vi "Main.vi"(8 "error in":errorcluster, 11 "System Monitor UI in":refnum<class "System Monitor UI.lvclass">) -> (0 "error out":errorcluster, 3 "System Monitor UI out":refnum<class "System Monitor UI.lvclass">)   [LabVIEW 2017, in "System Monitor UI.lvclass"]
doc: "The <b>Queued Message Handler</b> of the Worker that owns this VI."
uses:
  System Monitor UI.lvclass
  C:/Program Files (x86)/National Instruments/LabVIEW 2017/vi.lib/addons/_Workers/Library/Classes/Worker/Worker.lvclass
  Initialization Data.ctl
  Response Cases.ctl
  System Monitor UI.lvclass/System Monitor UI.ctl
  rwr_Get Main VI Ref.ctl
  rwr_Get Main VI Ref Reply.ctl
  rqp_Update cRIO System Data.ctl
  Shared/System Health Data.ctl
  <vilib>/addons/_Workers/Library/Classes/Message Queue/Message Queue.lvclass
panel:
  out "Total Virtual Memory (MB)":u32
  out "Total Physical Memory (MB)":u32
  out "Primary Hard Drive Capacity (MB)":u32
  out "Primary Hard Drive Available (MB)":dbl
  out "Hard Drive Space Used (%)":dbl(slide) scale=0.0..100.0
  out "Memory":dbl[][](graph)
  out "CPUs":u32[][](graph)
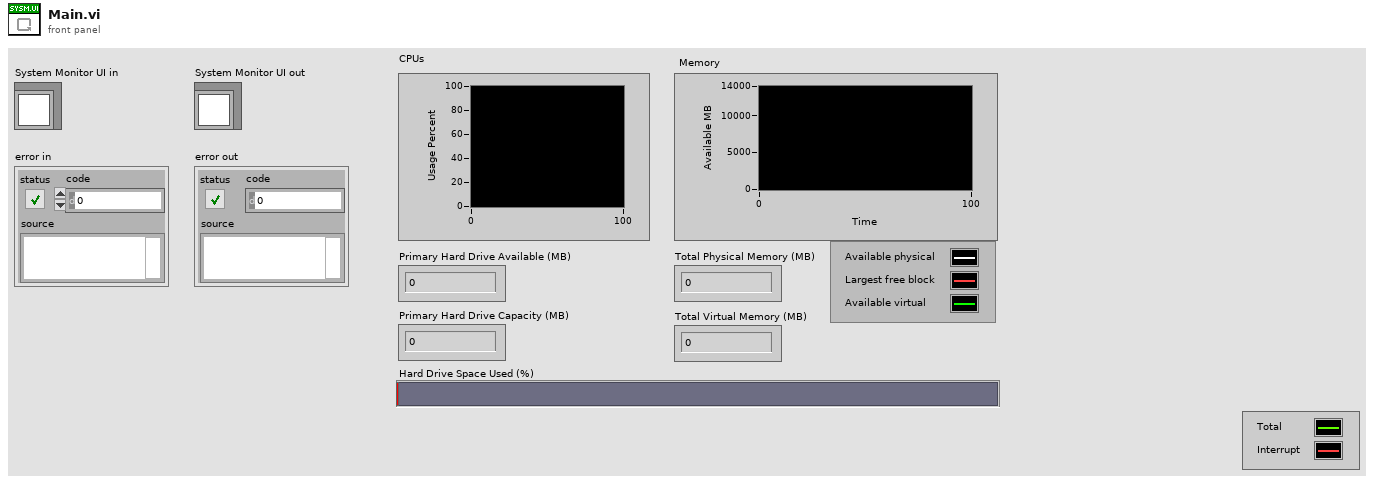
[diagram p1: front panel]
types:
  T1 = typedef "System Monitor UI.lvclass/Initialization Data.ctl" = cluster{"Response Cases":T2}
  T2 = typedef "System Monitor UI.lvclass/Response Cases.ctl" = cluster{"Placeholder - Can be deleted":string}
  T3 = typedef "System Monitor UI.lvclass/rwr_Get Main VI Ref Reply.ctl" = cluster{"Main VI Ref":refnum<vi>}
  T4 = typedef "System Monitor UI.lvclass/rwr_Get Main VI Ref.ctl" = cluster{"String":string}
  T5 = typedef "System Health Data.ctl" = cluster{"CPUs":u32[][], "Memory":dbl[][], "Hard Drive Space Used (%)":dbl, "Primary Hard Drive Available (MB)":dbl, "Primary Hard Drive Capacity (MB)":u32, "Total Physical Memory (MB)":u32, "Total Virtual Memory (MB)":u32}
  T6 = typedef "System Monitor UI.lvclass/rqp_Update cRIO System Data.ctl" = cluster{"Data as String":string}
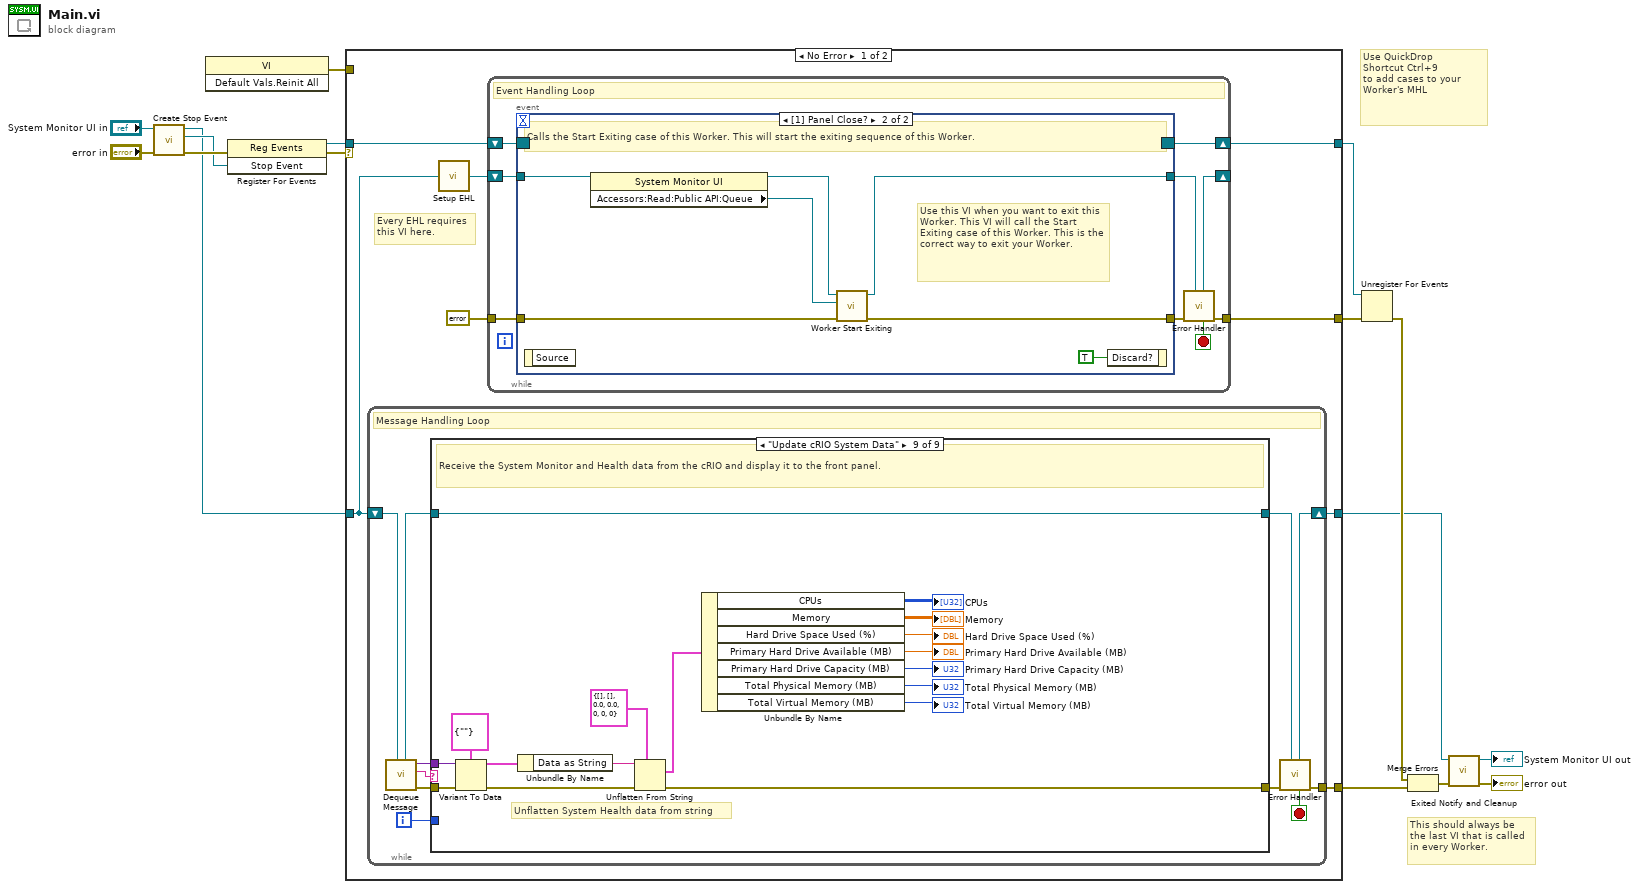
[diagram p0: block diagram]
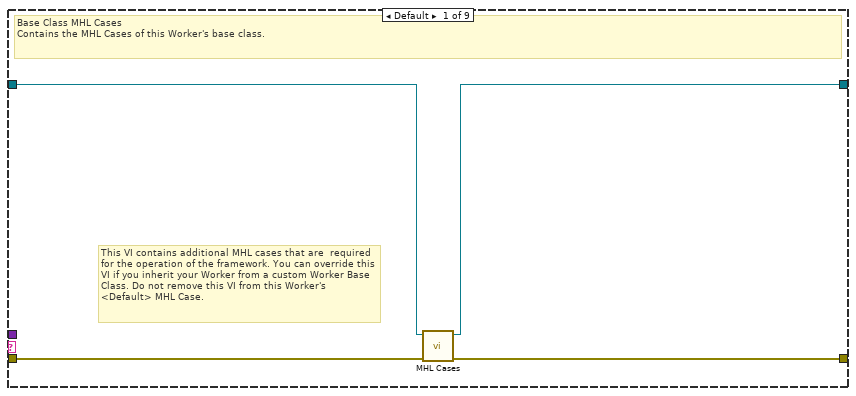
[diagram p2: hidden frame]
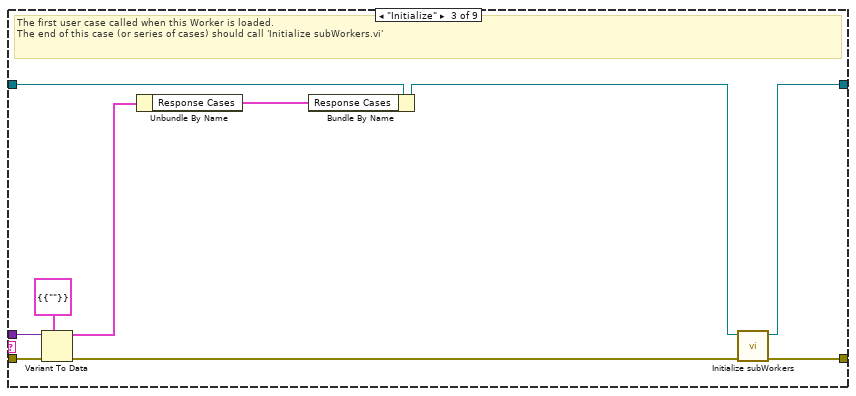
[diagram p4: hidden frame]
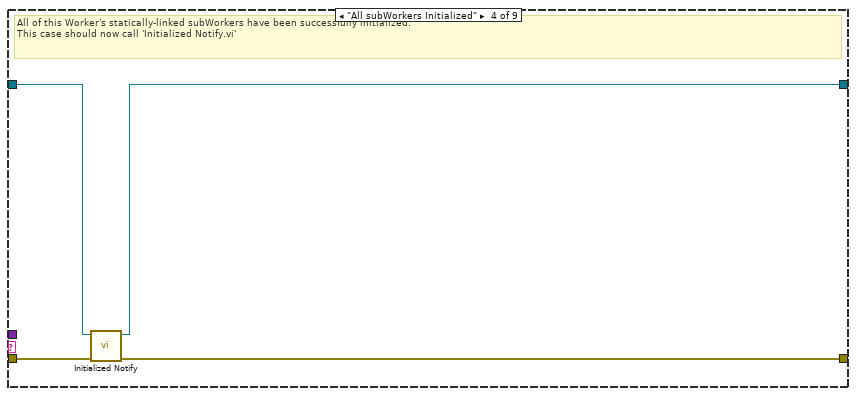
[diagram p5: hidden frame]
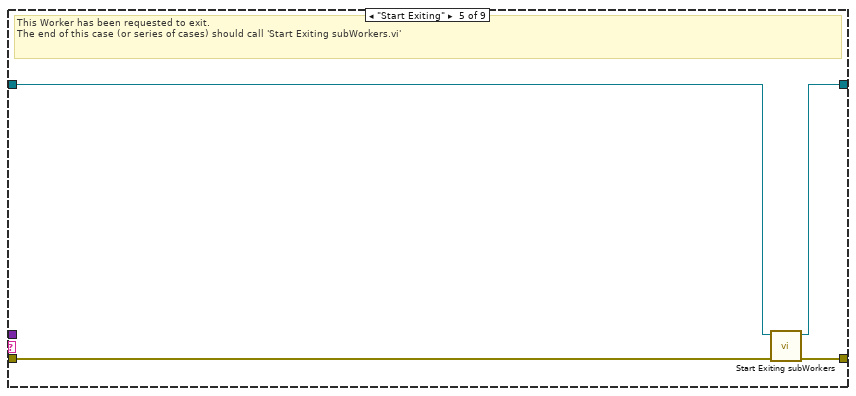
[diagram p6: hidden frame]
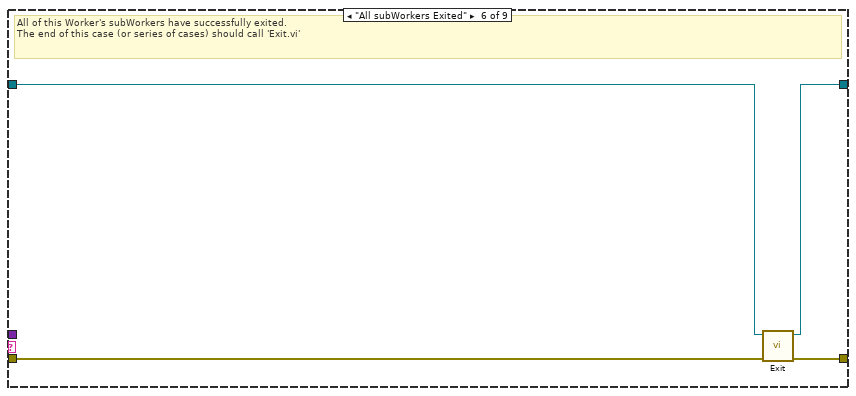
[diagram p7: hidden frame]
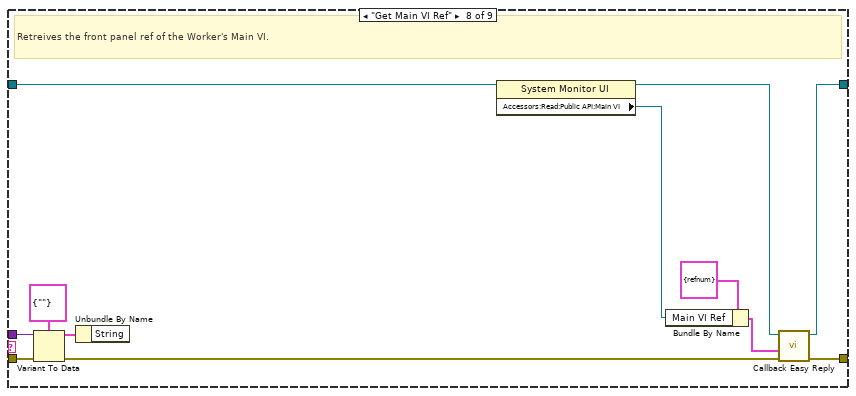
[diagram p9: hidden frame]
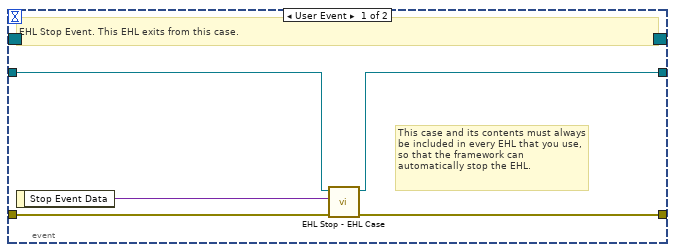
[diagram p10: hidden frame]
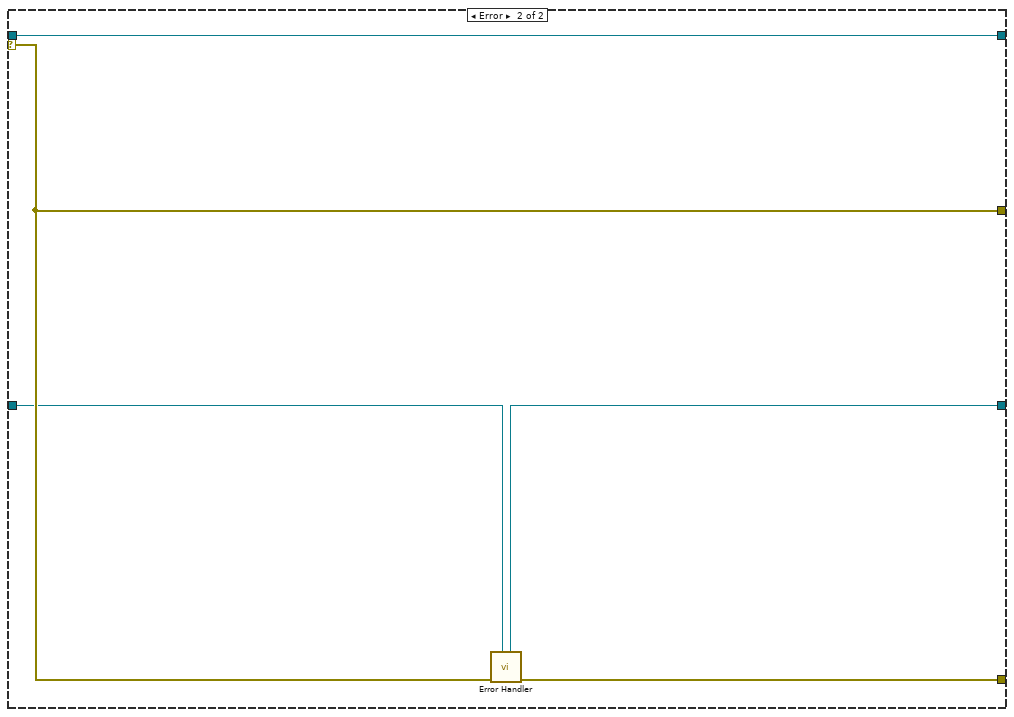
[diagram p11: hidden frame]
diagram:
  # "Use QuickDrop\nShortcut Ctrl+9\nto add cases to your\nWorker's MHL"
  # "This should always be the last VI that is called in every Worker."
  n1 = call-dynamic "Create Stop Event.vi"("error in"="error in", "Worker"="System Monitor UI in") -> ("error out"=w11:errorcluster, "Stop Event"=w8:refnum<user-event>, "Worker out"=w5:refnum<class "System Monitor UI.lvclass">)  [unwired: 7 in]
  n2 = invoke class="VI" method="Default Vals.Reinit All"() -> (error out=w1:errorcluster)  [unwired: 3 in, 2 out]
  n3 = register-events(error in=w11, w8) -> (reference out=w10:refnum<event-registration>, error out=w2:errorcluster)  [unwired: 1 in]
  n4 = case shown="No Error" w2 {
    tunnel: w5 -> [w19 w117]
    tunnel: [w17 w118] -> w9
    tunnel: w10 -> [w24 w119]
    tunnel: [w21 w120] -> w15
    tunnel: [w23 w119] -> w14
    tunnel: [w18 w116] -> w12
    selector: w2 -> [_ w120]
    tunnel: w1 -> [_ _]
    frame No Error {
      # "Every EHL requires\nthis VI here."
      n5 = while {
        shift-right: [w33] -> w18
        shift-left: w19 -> [w35]
        tunnel: [w34] -> w17
        i -> [w26]
        stop <- w27 stop-if-true
        # "Message Handling Loop"
        n6 = call-dynamic "Dequeue Message.vi"("Worker"=w35) -> ("error out"=w32:errorcluster, "Case out"=w28:string, "Data out"=w25:variant, "Worker out"=w30:refnum<class "System Monitor UI.lvclass">)  [unwired: 6 in, 1 out]
        n7 = case "Worker MHL Case Structure (DO NOT CHANGE LABEL NAME)" shown="\"Update cRIO System Data\"" w28 {
          tunnel: w32 -> [w39 w40 w49 w53 w56 w63 w65 w77 w93]
          tunnel: [w38 w40 w51 w52 w59 w62 w65 w72 w88] -> w31
          tunnel: w30 -> [w37 w41 w48 w55 w57 w61 w64 w70 w94]
          tunnel: [w36 w41 w50 w54 w58 w60 w64 w71 w94] -> w29
          tunnel: w26 -> [_ _ _ _ _ _ _ _ _]
          tunnel: w25 -> [_ _ w46 _ _ _ _ w74 w90]
          frame Default {
            # "This VI contains additional MHL cases that are  required for the operation of the framework. You can override this VI if you inherit your Worker from a custom Worker Base Class. Do not remove this VI from this Worker's <Default> MHL Case."
            # "Base Class MHL Cases\nContains the MHL Cases of this Worker's base class."
            n8 = call-dynamic "MHL Cases.vi"("error in"=w39, "Worker in"=w37) -> ("error out"=w38:errorcluster, "Worker out"=w36:refnum<class "System Monitor UI.lvclass">)  [unwired: 8 in]
          }
          frame "------------ FRAMEWORK CASES -----------" {
            # "Start of Workers Framework Cases"
          }
          frame "Initialize" {
            # "The first user case called when this Worker is loaded.\nThe end of this case (or series of cases) should call 'Initialize subWorkers.vi'"
            n9 = Variant To Data(error in=w49, type=T1 {"Response Cases"={"Placeholder - Can be deleted"=""}} ("Initialization Data"), Variant=w46) -> (data=w44:T1, error out=w47:errorcluster)
            n10 = Unbundle By Name(w44) -> ("Response Cases"=w43:T2)
            n11 = Bundle By Name(cluster=w48, "Response Cases"=w43) -> (w45:refnum<class "System Monitor UI.lvclass">)
            n12 = call-dynamic "Initialize subWorkers.vi"("error in"=w47, "Worker"=w45) -> ("error out"=w51:errorcluster, "dup Worker out"=w50:refnum<class "System Monitor UI.lvclass">)  [unwired: 8 in]
          }
          frame "All subWorkers Initialized" {
            # "All of this Worker's statically-linked subWorkers have been successfully initialized.\nThis case should now call 'Initialized Notify.vi'"
            n13 = call-dynamic "Initialized Notify.vi"("error in"=w53, "Worker"=w55) -> ("error out"=w52:errorcluster, "dup Worker out"=w54:refnum<class "System Monitor UI.lvclass">)  [unwired: 8 in]
          }
          frame "Start Exiting" {
            # "This Worker has been requested to exit. \nThe end of this case (or series of cases) should call 'Start Exiting subWorkers.vi'"
            n14 = call-dynamic "Start Exiting subWorkers.vi"("error_in"=w56, "Worker"=w57) -> ("error out"=w59:errorcluster, "dup Worker out"=w58:refnum<class "System Monitor UI.lvclass">)  [unwired: 8 in]
          }
          frame "All subWorkers Exited" {
            # "All of this Worker's subWorkers have successfully exited. \nThe end of this case (or series of cases) should call 'Exit.vi'"
            n15 = call-dynamic "Exit.vi"("error_in"=w63, "Worker"=w61) -> ("error out"=w62:errorcluster, "dup Worker out"=w60:refnum<class "System Monitor UI.lvclass">)  [unwired: 8 in]
          }
          frame "------------- PUBLIC API CASES -------------" {
            # "Start of Workers Public API Cases"
          }
          frame "Get Main VI Ref" {
            # "Retreives the front panel ref of the Worker's Main VI."
            n16 = Variant To Data(error in=w77, type=T4 {"String"=""} ("Data"), Variant=w74) -> (data=w73:T4, error out=w76:errorcluster)
            n17 = Unbundle By Name(w73) -> ()  [unwired: 1 out]
            n18 = property class="System Monitor UI"(reference=w70) -> (reference out=w68:refnum<class "System Monitor UI.lvclass">, "Accessors:Read:Public API:Main VI"=w66:refnum<vi>)  [unwired: 1 in, 1 out]
            n19 = Bundle By Name(cluster=T3 {"Main VI Ref"=refnum} ("Reply Data"), "Main VI Ref"=w66) -> (w67:T3)
            n20 = call-dynamic "Callback Easy Reply.vi"("error in"=w76, "Data"=w67, "Worker"=w68) -> ("error out"=w72:errorcluster, "dup Worker out"=w71:refnum<class "System Monitor UI.lvclass">)  [unwired: 7 in]
          }
          frame "Update cRIO System Data" {
            # "Unflatten System Health data from string"
            # "Receive the System Monitor and Health data from the cRIO and display it to the front panel."
            n21 = Variant To Data(error in=w93, type=T6 {"Data as String"=""} ("Data"), Variant=w90) -> (data=w89:T6, error out=w92:errorcluster)
            n22 = Unbundle By Name(w89) -> ("Data as String"=w87:string)
            n23 = Unflatten From String(type=T5 {"CPUs"=[], "Memory"=[], "Hard Drive Space Used (%)"=0.0, "Primary Hard Drive Available (MB)"=0.0, "Primary Hard Drive Capacity (MB)"=0, "Total Physical Memory (MB)"=0, "Total Virtual Memory (MB)"=0} ("System Health Data"), binary string=w87, error in (no error)=w92) -> (value=w85:T5, error out=w88:errorcluster)  [unwired: 2 in, 1 out]
            n24 = Unbundle By Name(w85) -> ("CPUs"=→"CPUs":u32[][], "Memory"=→"Memory":dbl[][], "Hard Drive Space Used (%)"=→"Hard Drive Space Used (%)":dbl, "Primary Hard Drive Available (MB)"=→"Primary Hard Drive Available (MB)":dbl, "Primary Hard Drive Capacity (MB)"=→"Primary Hard Drive Capacity (MB)":u32, "Total Physical Memory (MB)"=→"Total Physical Memory (MB)":u32, "Total Virtual Memory (MB)"=→"Total Virtual Memory (MB)":u32)
          }
        }
        n25 = call-dynamic "Error Handler.vi"("Worker"=w29, "error_in"=w31) -> ("error out"=w34:errorcluster, "Stop Loop"=w27:bool, "Worker out"=w33:refnum<class "System Monitor UI.lvclass">)  [unwired: 7 in]
      }
      n26 = call-dynamic "Setup EHL.vi"("Worker"=w19) -> ("Worker out"=w20:refnum<class "System Monitor UI.lvclass">)  [unwired: 14 in]
      n27 = while "Event Handling Loop" {
        shift-right: [w103] -> w23
        shift-left: w24 -> [w102]
        tunnel: [w98] -> w21
        tunnel: errorcluster {"status"=FALSE, "code"=0, "source"=""} ("error constant") -> [w100]
        shift-right: [w96] -> _
        shift-left: w20 -> [w101]
        stop <- w95 stop-if-true
        # "Event Handling Loop"
        n28 = event shown="[1] Panel Close?" {
          selector: w102 -> [_ _]
          dyn-events: [_ _] -> w103
          timeout: _ -> [_ _]
          tunnel: [w107 w114] -> w99
          tunnel: w100 -> [w108 w113]
          tunnel: w101 -> [w106 w112]
          tunnel: [w105 w111] -> w97
          event User Event {
            # "This case and its contents must always be included in every EHL that you use, so that the framework can automatically stop the EHL."
            # "EHL Stop Event. This EHL exits from this case."
            n29 = event-data() -> ("Stop Event Data"=w104:variant)  [unwired: 1 in]
            n30 = call-dynamic "EHL Stop - EHL Case.vi"("error in"=w108, "Stop Event Data"=w104, "Worker"=w106) -> ("error out"=w107:errorcluster, "Worker out"=w105:refnum<class "System Monitor UI.lvclass">)  [unwired: 7 in]
          }
          event Panel Close? {
            # "Use this VI when you want to exit this Worker. This VI will call the Start Exiting case of this Worker. This is the correct way to exit your Worker."
            # "Calls the Start Exiting case of this Worker. This will start the exiting sequence of this Worker."
            n31 = event-data() -> ()  [unwired: 1 in, 1 out]
            n32 = property class="System Monitor UI"(reference=w112) -> (reference out=w110:refnum<class "System Monitor UI.lvclass">, "Accessors:Read:Public API:Queue"=w109:refnum<class "Message Queue.lvclass">)  [unwired: 1 in, 1 out]
            n33 = call-dynamic "Worker Start Exiting.vi"("error_in"=w113, "Message Queue"=w109, "Worker"=w110) -> ("error out"=w114:errorcluster, "dup Worker out"=w111:refnum<class "System Monitor UI.lvclass">)  [unwired: 7 in]
            n34 = event-data("Discard?"=TRUE) -> ()  [unwired: 1 in, 1 out]
          }
        }
        n35 = call-dynamic "Error Handler.vi"("Worker"=w97, "error_in"=w99) -> ("error out"=w98:errorcluster, "Stop Loop"=w95:bool, "Worker out"=w96:refnum<class "System Monitor UI.lvclass">)  [unwired: 7 in]
      }
    }
    frame Error {
      n36 = call-dynamic "Error Handler.vi"("Worker"=w117, "error_in"=w120) -> ("error out"=w118:errorcluster, "Worker out"=w116:refnum<class "System Monitor UI.lvclass">)  [unwired: 7 in, 1 out]
    }
  }
  n37 = Unregister For Events(event registration refnum=w14, error in=w15) -> (error out=w16:errorcluster)
  n38 = Merge Errors(w16, w9) -> (w13:errorcluster)
  n39 = call-dynamic "Exited Notify and Cleanup.vi"("error_in"=w13, "Worker"=w12) -> ("error out"=→"error out":errorcluster, "dup Worker out"=→"System Monitor UI out":refnum<class "System Monitor UI.lvclass">)  [unwired: 8 in]
